vi "Close.vi"(8 "error in (no error)":errorcluster, 11 "IConnection in":refnum<class "IConnection.lvclass">) -> (0 "error out":errorcluster)   [LabVIEW 2019, in "Network Interface.lvlib" / "IConnection.lvclass"]
uses:
  <vilib>/gpm_packages/@cs/Network-Sink/Source/Network Interface/IConnection/IConnection.lvclass
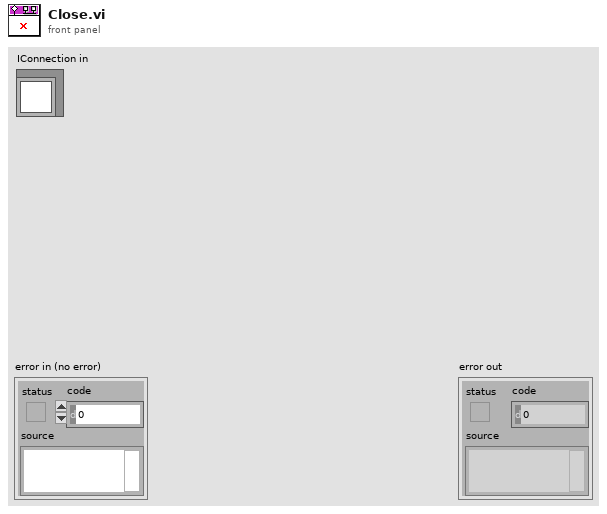
[diagram p1: front panel]
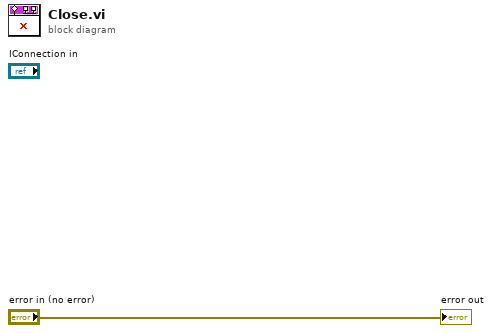
[diagram p0: block diagram]
diagram:
  "error out" <- "error in (no error)"
